vi "tearDown.vi"(8 "error in":errorcluster, 11 "reference in":refnum<class "Create Execution Unit.lvclass">) -> (0 "error out":errorcluster, 3 "reference out":refnum<class "Create Execution Unit.lvclass">)   [LabVIEW 2020, in "Create Execution Unit.lvclass"]
doc: "tearDown runs after the test method has completed. Use this method to clean up any operations or references that were opened by setUp or the test method. Unit tests should be independent of other unit tests so this VI should ensure that the next test can run in a 'clean' test environment."
uses:
  Create Execution Unit.lvclass
  C:/Users/nitest/Desktop/Git 2020/niveristand-custom-device-testing-tools/VeriStandScriptingTestCase/VeriStandScriptingTestCase.lvclass
  niveristand-custom-device-testing-tools/VeriStandScriptingTestCase/VeriStandScriptingTestCase.lvclass
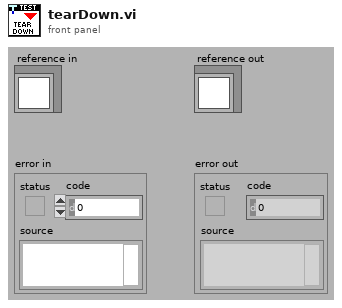
[diagram p1: front panel]
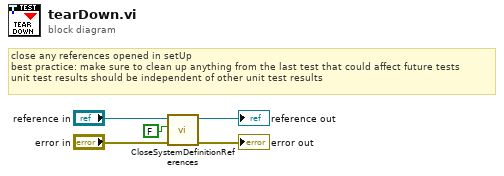
[diagram p0: block diagram]
diagram:
  # "close any references opened in setUp\nbest practice: make sure to clean up anything from the last test that could affect future tests\nunit test results should be independent of other unit test results"
  n1 = call "CloseSystemDefinitionReferences.vi"("error in"="error in", "Delete Sysdef? (F)"=FALSE, "VeriStandScriptingTestCase in"="reference in") -> ("error out"=→"error out":errorcluster, "VeriStandScriptingTestCase out"=→"reference out":refnum<class "Create Execution Unit.lvclass">)  [unwired: 7 in]
